vi "Map.vi"(2 "Value In":variant, 3 "Name":string, 4 "Map In":variant) -> (0 "Value Out":variant, 1 "Map Out":variant)   [LabVIEW 2014]
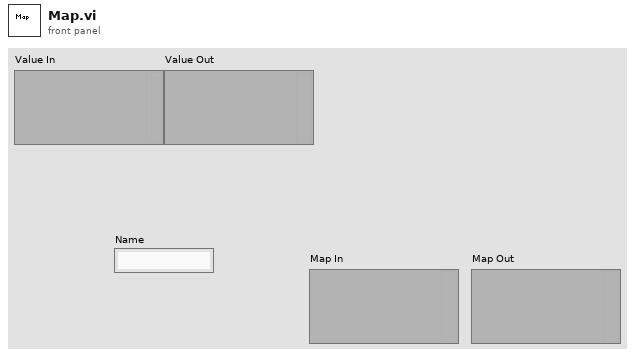
[diagram p1: front panel]
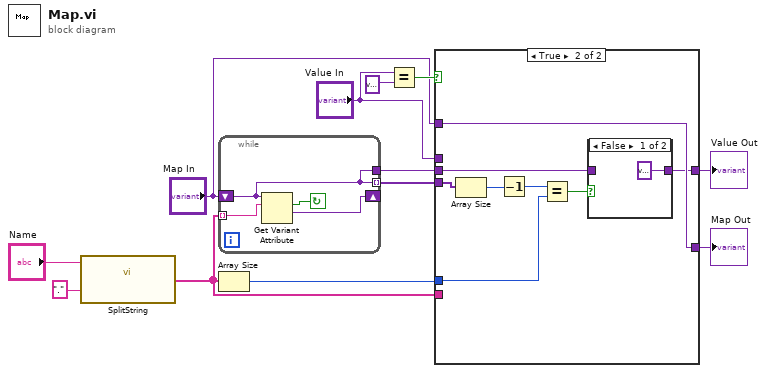
[diagram p0: block diagram]
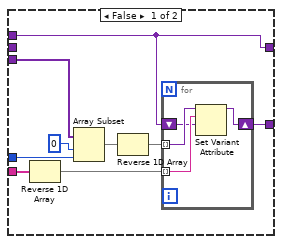
[diagram p2: hidden frame]
diagram:
  n1 = call "SplitString.vi"("Delimeter"=".", "Name"="Name") -> ("Array"=w2:string[])
  n2 = while {
    tunnel: w2 -> [w16] mode=indexing
    shift-right: [w15] -> _
    shift-left: "Map In" -> [w13]
    tunnel: [w13] -> w5 mode=indexing
    tunnel: [w13] -> w3
    stop <- w14 continue-if-true
    n3 = Get Variant Attribute(Variant=w13, name=w16) -> (found=w14:bool, value=w15:variant)  [unwired: 2 in, 2 out]
  }
  n4 = Array Size(array=w2) -> (size(s)=w1:i32)
  n5 = Equal?(x="Value In", y=variant ("Value In")) -> (x = y?=w9:bool)
  n6 = case shown="True" w9 {
    tunnel: [w22 w33] -> w8
    tunnel: "Map In" -> [_ w37]
    tunnel: [w23 w37] -> w6
    tunnel: w5 -> [w20 w36]
    tunnel: w2 -> [w25 _]
    tunnel: "Value In" -> [w22 _]
    tunnel: w3 -> [_ w32]
    tunnel: w1 -> [w19 w35]
    frame False {
      n7 = Reverse 1D Array(array=w25) -> (reversed array=w24:string[])
      n8 = Array Subset(array=w20, index=0, length=w19) -> (w18:variant[])
      n9 = Reverse 1D Array(array=w18) -> (reversed array=w17:variant[])
      n10 = for {
        tunnel: w24 -> [w28] mode=indexing
        tunnel: w17 -> [w29] mode=indexing
        shift-right: [w26] -> w23
        shift-left: w22 -> [w27]
        n11 = Set Variant Attribute(Variant=w29, name=w28, value=w27) -> (Variant out=w26:variant)  [unwired: 1 in, 2 out]
      }
    }
    frame True {
      n12 = Array Size(array=w36) -> (size(s)=w31:i32)
      n13 = Decrement(x=w31) -> (x-1=w30:i32)
      n14 = Equal?(x=w30, y=w35) -> (x = y?=w34:bool)
      n15 = case shown="False" w34 {
        tunnel: [variant ("Value In") w39] -> w33
        tunnel: w32 -> [_ w39]
        frame False {
        }
        frame True {
        }
      }
    }
  }
  "Map Out" <- w6
  "Value Out" <- w8
